vi "Distribute Panel Objects.vi"(8 "error in (no error)":errorcluster, 10 "Distribution Type":T1, 11 "Panel Objects in":refnum<class "Panel Object.lvclass">[](array[class])) -> (0 "error out":errorcluster, 3 "Panel Objects out":refnum<class "Panel Object.lvclass">[](array[class]))   [LabVIEW 2017, in "Panel Object.lvclass"]
uses:
  Panel Object.lvclass
  Distribution Type--Enum.ctl
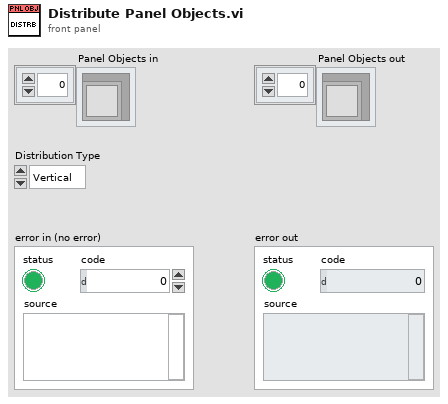
[diagram p1: front panel]
types:
  T1 = typedef "Distribution Type--Enum.ctl" = enum16{"Vertical", "Horizontal"}
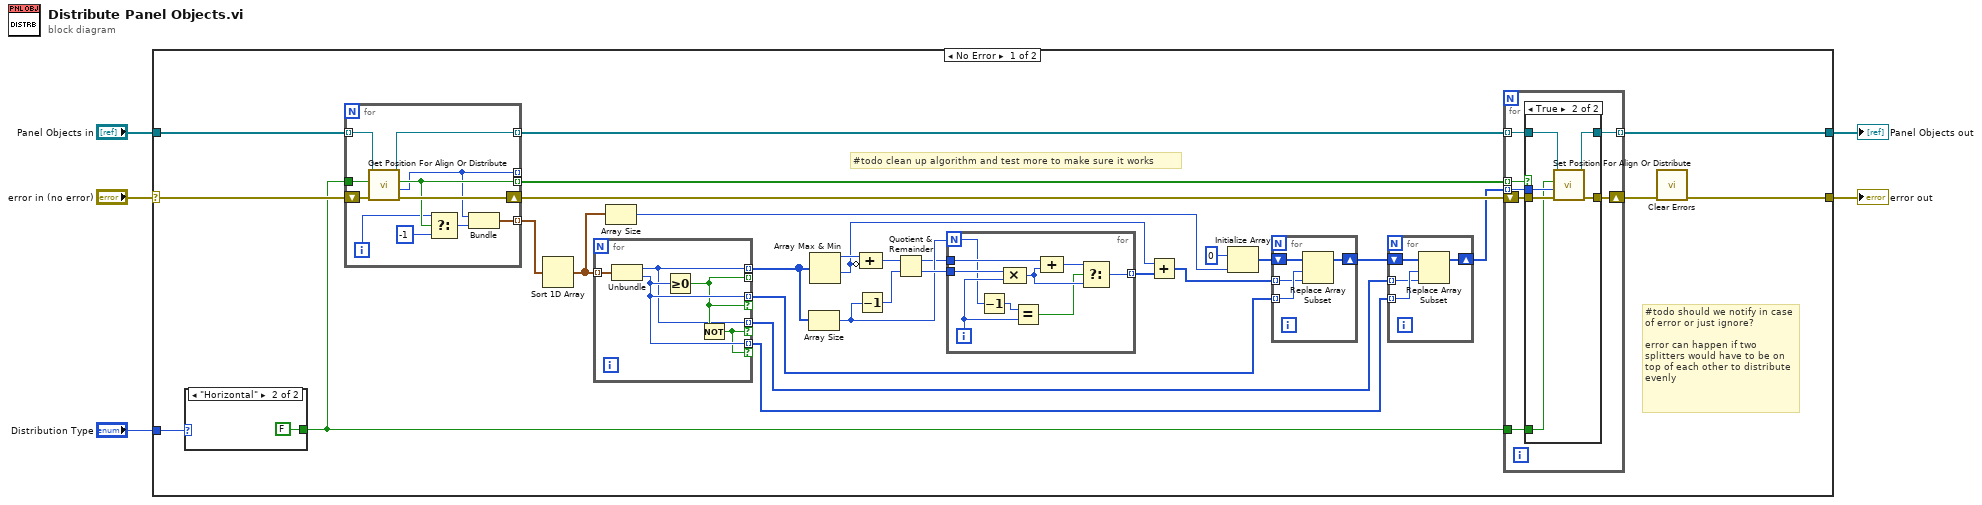
[diagram p0: block diagram]
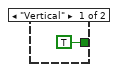
[diagram p2: hidden frame]
diagram:
  n1 = case shown="No Error" "error in (no error)" {
    selector: "error in (no error)" -> [w29 w86]
    tunnel: [w34 w87] -> w5
    tunnel: "Panel Objects in" -> [w30 w87]
    tunnel: [w28 w86] -> w2
    tunnel: "Distribution Type" -> [w26 _]
    frame No Error {
      # "#todo clean up algorithm and test more to make sure it works"
      # "#todo should we notify in case of error or just ignore?\n\nerror can happen if two splitters would have to be on top of each other to distribute evenly"
      n2 = case shown="\"Horizontal\"" w26 {
        tunnel: [TRUE FALSE] -> w27
        frame "Vertical" {
        }
        frame "Horizontal" {
        }
      }
      n3 = for {
        shift-right: [w63] -> w31
        shift-left: w29 -> [w66]
        tunnel: w30 -> [w65] mode=indexing
        tunnel: [w64] -> w33 mode=indexing
        tunnel: [w59] -> _ mode=indexing
        tunnel: [w61] -> w35 mode=indexing
        tunnel: w27 -> [w62]
        tunnel: [w56] -> w14 mode=indexing
        i -> [w58]
        n4 = call-dynamic "Get Position For Align Or Distribute.vi"("Error In"=w66, "Vertical? (F: Horizontal)"=w62, "Panel Object in"=w65) -> ("Error Out"=w63:errorcluster, "Position"=w59:i32, "Applicable?"=w61:bool, "Panel Object out"=w64:refnum<class "Panel Object.lvclass">)  [unwired: 5 in]
        n5 = Select(t=w58, s=w61, f=-1) -> (s? t:f=w57:i32)
        n6 = Bundle("Position"=w59, "f"=w57) -> (w56:cluster{"Position":i32, "f":i32})  [unwired: 1 in]
      }
      n7 = Sort 1D Array(array=w14) -> (sorted array=w13:cluster{"Position":i32, "f":i32}[])
      n8 = for {
        tunnel: w13 -> [w53] mode=indexing
        tunnel: [w50] -> w12 mode=indexing if=w51
        tunnel: [w51] -> _ mode=indexing
        tunnel: [w52] -> w11 mode=indexing if=w51
        tunnel: [w52] -> w7 mode=indexing if=w49
        tunnel: [w50] -> w8 mode=indexing if=w49
        n9 = Unbundle(w53) -> ("Position"=w50:i32, "f"=w52:i32)
        n10 = Greater Or Equal To 0?(x=w52) -> (x >= 0?=w51:bool)
        n11 = Not(x=w51) -> (.not. x?=w49:bool)
      }
      n12 = Array Size(array=w13) -> (size(s)=w17:i32)
      n13 = Array Size(array=w12) -> (size(s)=w21:i32)
      n14 = Array Max & Min(array=w12) -> (max value=w25:i32, min value=w18:i32)  [unwired: 2 out]
      n15 = Decrement(x=w21) -> (x-1=w23:i32)
      n16 = Compound Arithmetic op=ADD(w25, invert w18) -> (w24:i32)
      n17 = Quotient & Remainder(x=w24, y=w23) -> (x-y*floor(x/y)=w20:i32, floor(x/y)=w22:i32)
      n18 = for {
        N: w21 -> [w42]
        tunnel: w22 -> [w48]
        tunnel: w20 -> [w46]
        tunnel: [w40] -> w19 mode=indexing
        i -> [w47]
        n19 = Decrement(x=w42) -> (x-1=w41:i32)
        n20 = Compound Arithmetic op=MULTIPLY(w48, w47) -> (w45:i32)
        n21 = Equal?(x=w41, y=w47) -> (x = y?=w43:bool)
        n22 = Compound Arithmetic op=ADD(w46, w45) -> (w44:i32)
        n23 = Select(t=w44, s=w43, f=w45) -> (s? t:f=w40:i32)
      }
      n24 = Add(x=w18, y=w19) -> (x+y=w10:i32[])
      n25 = Initialize Array(0, w17) -> (w15:i32[])
      n26 = for {
        tunnel: w11 -> [w68] mode=indexing
        shift-right: [w69] -> w9
        shift-left: w15 -> [w70]
        tunnel: w10 -> [w67] mode=indexing
        n27 = Replace Array Subset(array=w70, new element=w67, index=w68) -> (w69:i32[])
      }
      n28 = for {
        tunnel: w7 -> [w37] mode=indexing
        shift-right: [w38] -> w6
        shift-left: w9 -> [w39]
        tunnel: w8 -> [w36] mode=indexing
        n29 = Replace Array Subset(array=w39, new element=w36, index=w37) -> (w38:i32[])
      }
      n30 = for {
        tunnel: w6 -> [w77] mode=indexing
        shift-right: [w75] -> w32
        shift-left: w31 -> [w76]
        tunnel: w33 -> [w74] mode=indexing
        tunnel: [w73] -> w34 mode=indexing
        tunnel: w35 -> [w72] mode=indexing
        tunnel: w27 -> [w71]
        n31 = case shown="True" w72 {
          tunnel: w77 -> [_ w85]
          tunnel: w76 -> [w78 w84]
          tunnel: [w78 w83] -> w75
          tunnel: w74 -> [w79 w82]
          tunnel: [w79 w81] -> w73
          tunnel: w71 -> [_ w80]
          frame False {
          }
          frame True {
            n32 = call-dynamic "Set Position For Align Or Distribute.vi"("Error In"=w84, "Position"=w85, "Vertical? (F: Horizontal)"=w80, "Panel Object in"=w82) -> ("Error Out"=w83:errorcluster, "Panel Object out"=w81:refnum<class "Panel Object.lvclass">)  [unwired: 6 in]
          }
        }
      }
      n33 = call <vilib>:"Clear Errors.vi"("error in (no error)"=w32) -> ("error out"=w28:errorcluster)  [unwired: 5 in, 1 out]
    }
    frame Error {
    }
  }
  "Panel Objects out" <- w5
  "error out" <- w2
